vi "Init Alternative.vi"(5 "Label":string, 8 "error in (no error)":errorcluster, 10 "Items":refnum<class "IObject.lvclass">[](array[class])) -> (0 "error out":errorcluster, 3 "Viewport out":refnum<class "Alternative.lvclass">)   [LabVIEW 2021, in "Alternative.lvclass"]
doc: "Copyright 2018, Wiebe Walstra, wiebe@carya.nl."
uses:
  Alternative.lvclass
  C:/Projects/Dynamic-Scaling/Dynamic Scaling/IContainer/IContainer.lvclass
  C:/Projects/Dynamic-Scaling/Dynamic Scaling/IObject.lvclass
  IObject.lvclass
  Alternative.lvclass/Alternative.ctl
  IContainer.lvclass
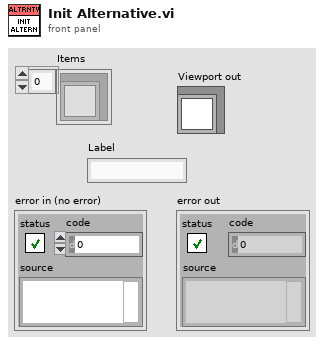
[diagram p1: front panel]
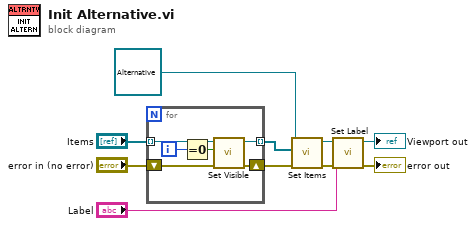
[diagram p0: block diagram]
diagram:
  n1 = for {
    tunnel: "Items" -> [w14] mode=indexing
    tunnel: [w13] -> w5 mode=indexing
    shift-right: [w15] -> w7
    shift-left: "error in (no error)" -> [w16]
    i -> [w11]
    n2 = Equal To 0?(x=w11) -> (x = 0?=w12:bool)
    n3 = call-dynamic "Set Visible.vi"("error in (no error)"=w16, "Show? [T]"=w12, "MMI Scaling in"=w14) -> ("error out"=w15:errorcluster, "MMI Scaling out"=w13:refnum<class "IObject.lvclass">)  [unwired: 7 in]
  }
  n4 = call "Set Items.vi"("error in (no error)"=w7, "Items"=w5, "IContainer in"=refnum<class "Alternative.lvclass"> refnum ("Viewport in")) -> ("error out"=w9:errorcluster, "IContainer out"=w3:refnum<class "Alternative.lvclass">)  [unwired: 7 in]
  n5 = call "Set Label.vi"("error in (no error)"=w9, "Label"="Label", "MMI Scaling in"=w3) -> ("error out"=→"error out":errorcluster, "MMI Scaling out"=→"Viewport out":refnum<class "Alternative.lvclass">)  [unwired: 7 in]
